vi "nifxpmath_ErrorCodes.vi"() -> ()   [LabVIEW 2017]
doc: "Defines error codes for the fxp math library. These error codes can be found in NI error code database under \"FXP Math Library\" product"
panel:
  in  "ExecutionModeErr":i32=-42802
  in  "InvConfigParaErr":i32=-42801
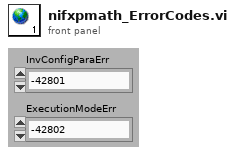
[diagram p1: front panel]
diagram:
